vi "Util-Query Unit Mode.vi"(8 "error in (no error)":errorcluster, 11 "VISA session":refnum<visa-resource-name>) -> (0 "error out":errorcluster, 2 "unit mode":u8[](array[ring]) items=["disabled or not installed", "V", "I", "common", "V pulse", "I pulse", "DV"], 3 "VISA resource name out":refnum<visa-resource-name>)   [LabVIEW 2016, in "Agilent 415X Series.lvlib"]
doc: "This VI queries the mode of each installed SMU and VMU."
uses:
  Agilent 415X Series.lvlib
panel:
  in  "unit mode":string[](array[string])=["D", "V", "I", "C"]
  in  "unit mode in":dbl[](array[ring]) items=["disabled or not installed", "V", "I", "common"]
  # "array index  unit name\n      0                VMU1\n      1                VMU2\n      2                SMU1\n      3                SMU2\n      4                SMU3\n      5                SMU4\n      6                SMU5\n      7                SMU6"
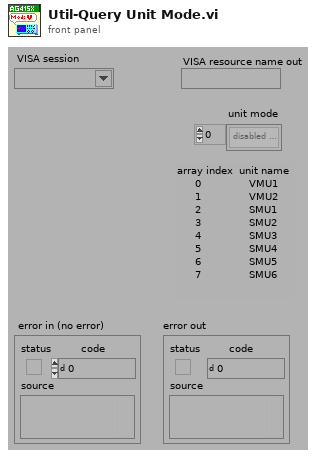
[diagram p1: front panel]
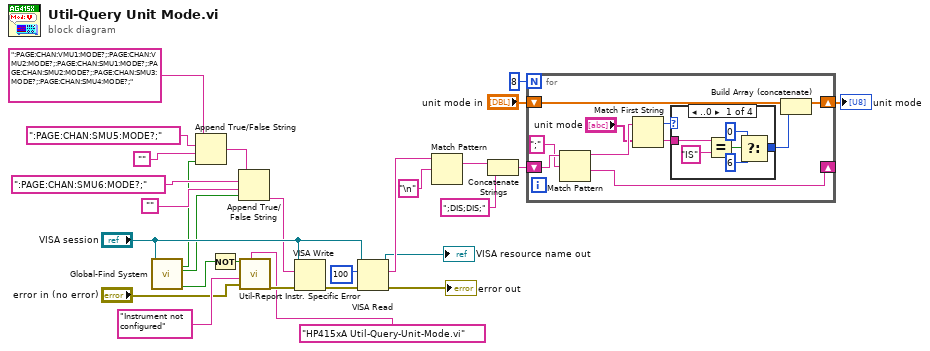
[diagram p0: block diagram]
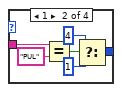
[diagram p2: hidden frame]
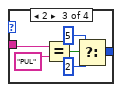
[diagram p3: hidden frame]
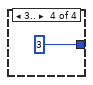
[diagram p4: hidden frame]
diagram:
  n1 = call "Global-Find System.vi"("VISA session"="VISA session") -> ("found"=w28:bool, "SMU6 present"=w5:bool, "SMU5 present"=w6:bool)  [unwired: 3 in, 5 out]
  n2 = Append True/False String(1:w6, 2:"", 3:":PAGE:CHAN:SMU5:MODE?;", 4:":PAGE:CHAN:VMU1:MODE?;:PAGE:CHAN:VMU2:MODE?;:PAGE:CHAN:SMU1:MODE?;:PAGE:CHAN:SMU2:MODE?;:PAGE:CHAN:SMU3:MODE?;:PAGE:CHAN:SMU4:MODE?;") -> (0:w23:string)
  n3 = Not(x=w28) -> (.not. x?=w27:bool)
  n4 = Append True/False String(1:w5, 2:"", 3:":PAGE:CHAN:SMU6:MODE?;", 4:w23) -> (0:w13:string)
  n5 = call "Util-Report Instr. Specific Error.vi"("source"="HP415xA Util-Query-Unit-Mode.vi", "error in (no error)"="error in (no error)", "error message"="Instrument not configured", "new error"=w27) -> ("error out"=w24:errorcluster)  [unwired: 6 in, 1 out]
  n6 = VISA Write(VISA resource name="VISA session", write buffer=w13, error in (no error)=w24) -> (error out=w15:errorcluster)  [unwired: 2 out]
  n7 = VISA Read(VISA resource name="VISA session", byte count=100, error in (no error)=w15) -> (VISA resource name out=→"VISA resource name out":refnum<visa-resource-name>, read buffer=w4:string, error out=→"error out":errorcluster)  [unwired: 1 out]
  n8 = Match Pattern(string=w4, regular expression="\n") -> (before substring=w2:string)  [unwired: 1 in, 3 out]
  n9 = Concatenate Strings(w2, ";DIS;DIS;") -> (w12:string)
  n10 = for {
    N: 8 -> [_]
    shift-right: [w31] -> _
    shift-left: w12 -> [w38]
    shift-right: [w33] -> w9
    shift-left: "unit mode in" -> [w35]
    n11 = Match Pattern(string=w38, regular expression=";") -> (before substring=w36:string, after substring=w31:string)  [unwired: 1 in, 2 out]
    n12 = Match First String(2:"unit mode", 3:w36) -> (0:w32:i32, 1:w30:string)
    n13 = case shown="..0" w32 {
      tunnel: w30 -> [w39 w45 w51 _]
      tunnel: [w42 w48 w54 3] -> w29
      frame ..0 {
        n14 = Equal?(x=w39, y="IS") -> (x = y?=w41:bool)
        n15 = Select(t=0, s=w41, f=6) -> (s? t:f=w42:i32)
      }
      frame 1 {
        n16 = Equal?(x=w45, y="PUL") -> (x = y?=w47:bool)
        n17 = Select(t=4, s=w47, f=1) -> (s? t:f=w48:i32)
      }
      frame 2 {
        n18 = Equal?(x=w51, y="PUL") -> (x = y?=w53:bool)
        n19 = Select(t=5, s=w53, f=2) -> (s? t:f=w54:i32)
      }
      frame 3.. {
      }
    }
    n20 = Build Array (concatenate)(w35, w29) -> (w33:dbl[])
  }
  "unit mode" <- w9
